vi "exif modifier.vi"(6 "Add info":T1(ring), 9 "modifier":string, 11 "input 1":path) -> (1 "error":string)   [LabVIEW 2023]
panel:
  # "exiftool \n-FileModifyDate \n-CreateDate \n-Make -Model \n-ProjectionType \n-ImageWidth \n-ImageHeight \n-Orientation \n-DateTimeOriginal"
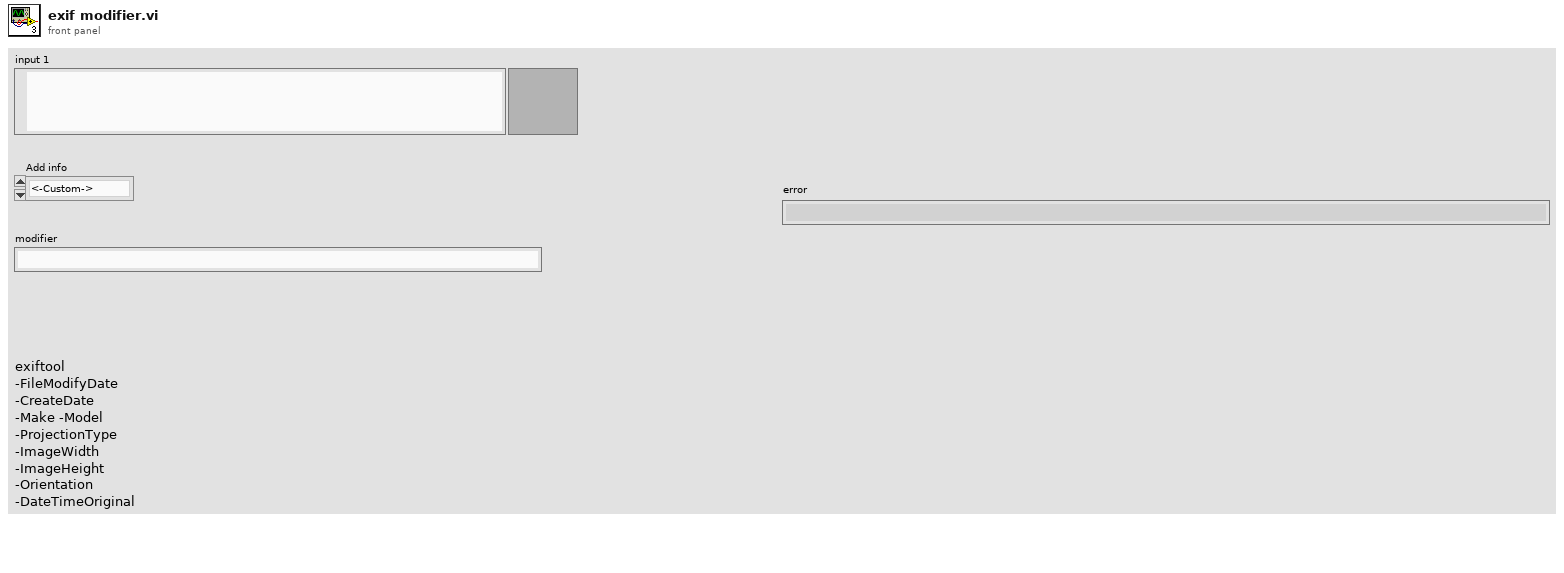
[diagram p1: front panel]
types:
  T1 = enum16{"<-Custom->", "Information", "Bills", "Medical"}
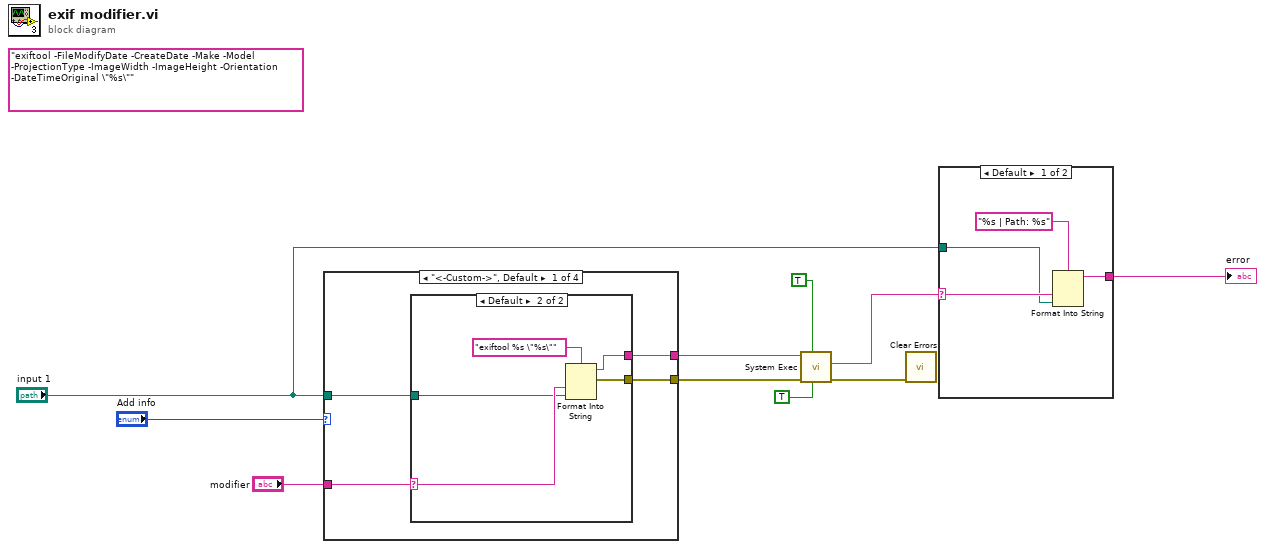
[diagram p0: block diagram]
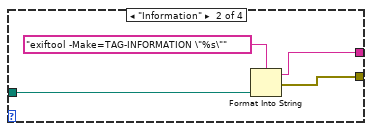
[diagram p3: hidden frame]
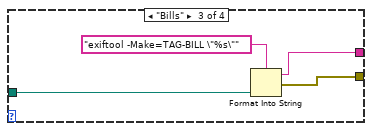
[diagram p4: hidden frame]
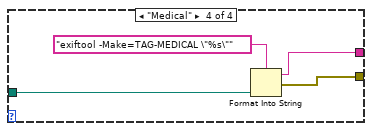
[diagram p5: hidden frame]
diagram:
  (unwired) "exiftool -FileModifyDate -CreateDate -Make -Model -ProjectionType -ImageWidth -ImageHeight -Orientation -DateTimeOriginal \"%s\"" ("command line")
  n1 = case shown="\"<-Custom->\", Default" "Add info" {
    tunnel: [w14 w23 w27 w31] -> w10
    tunnel: [w13 w22 w26 w30] -> w9
    tunnel: "modifier" -> [w12 _ _ _]
    tunnel: "input 1" -> [w11 w20 w24 w28]
    frame "<-Custom->", Default {
      n2 = case shown="Default" w12 {
        selector: w12 -> [_ w16]
        tunnel: [_ w19] -> w14
        tunnel: [_ w18] -> w13
        tunnel: w11 -> [_ w15]
        frame "" {
        }
        frame Default {
          n3 = Format Into String(format string="exiftool %s \"%s\"" ("command line"), w16, w15) -> (resulting string=w18:string, error out=w19:errorcluster)  [unwired: 2 in]
        }
      }
    }
    frame "Information" {
      n4 = Format Into String(format string="exiftool -Make=TAG-INFORMATION \"%s\"" ("command line"), w20) -> (resulting string=w22:string, error out=w23:errorcluster)  [unwired: 2 in]
    }
    frame "Bills" {
      n5 = Format Into String(format string="exiftool -Make=TAG-BILL \"%s\"" ("command line"), w24) -> (resulting string=w26:string, error out=w27:errorcluster)  [unwired: 2 in]
    }
    frame "Medical" {
      n6 = Format Into String(format string="exiftool -Make=TAG-MEDICAL \"%s\"" ("command line"), w28) -> (resulting string=w30:string, error out=w31:errorcluster)  [unwired: 2 in]
    }
  }
  n7 = call <vilib>:"System Exec.vi"("run minimized? (F)"=TRUE, "wait until completion? (T)"=TRUE, "error in (no error)"=w10, "command line"=w9) -> ("error out"=w7:errorcluster, "standard error"=w4:string)  [unwired: 4 in, 2 out]
  n8 = call <vilib>:"Clear Errors.vi"("error in (no error)"=w7) -> ()  [unwired: 5 in, 2 out]
  n9 = case shown="Default" w4 {
    selector: w4 -> [w35 w36]
    tunnel: [w33 w36] -> w3
    tunnel: "input 1" -> [w34 _]
    frame Default {
      n10 = Format Into String(format string="%s | Path: %s", w35, w34) -> (resulting string=w33:string)  [unwired: 2 in, 1 out]
    }
    frame "" {
    }
  }
  "error" <- w3
